vi "SQLite Example.vi"() -> ()   [LabVIEW 2011]
uses:
  State.ctl
  <vilib>/Analysis/NI_AALBase.lvlib
panel:
  out "Mean":dbl format="%0.2f"
  out "Failures":i32
  out "Voltage Waveform":dbl[](graph)
  # "Please refer to the readme in this project to make sure that the SQLite Engine is correctly installed on the real-time target"
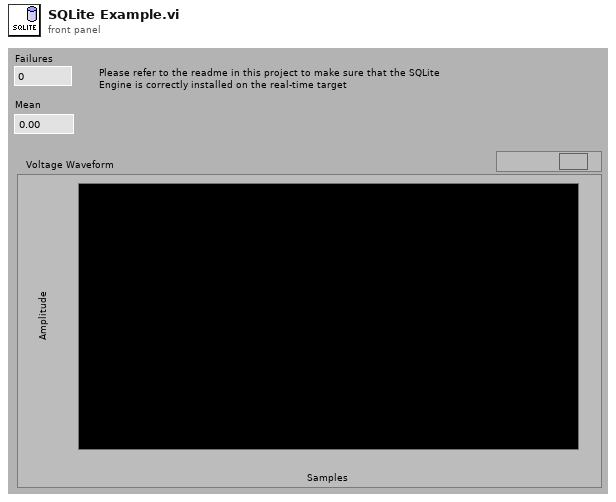
[diagram p1: front panel]
types:
  T1 = typedef "State.ctl" = enum16{"Empty Database", "Simulate Test", "Log DB", "Process DB", "Shutdown"}
  T2 = cluster{"RT State":T1, "Iteration":i32, "Record":cluster{"Iteration":i32, "Pass":bool, "Voltage":dbl, "log time":timestamp}}
  T3 = cluster{"Iteration":i32, "Pass":bool, "Voltage":dbl, "log time":timestamp}
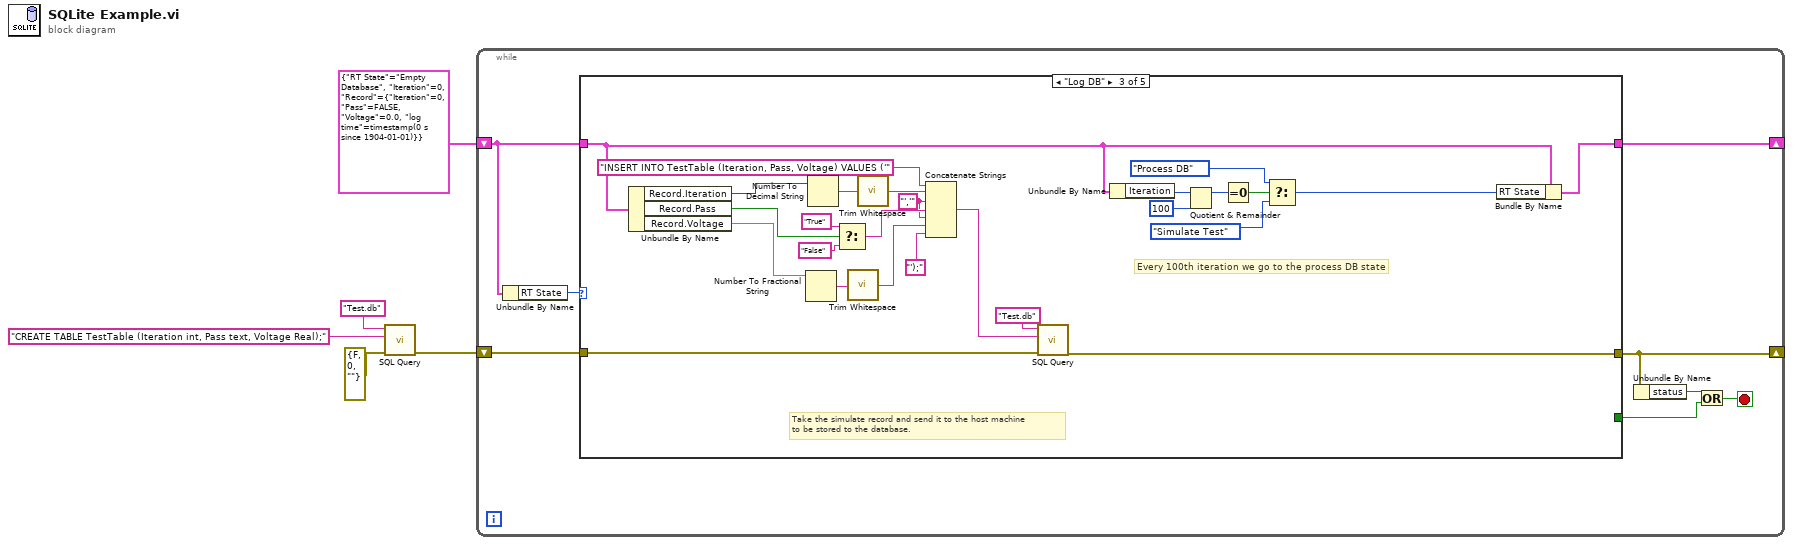
[diagram p0: block diagram]
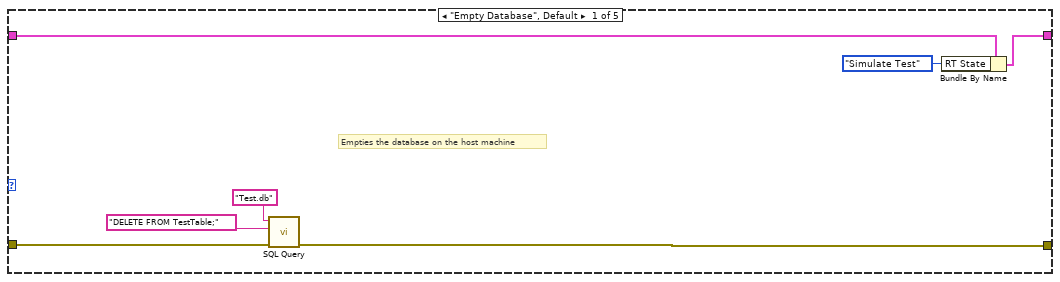
[diagram p2: hidden frame]
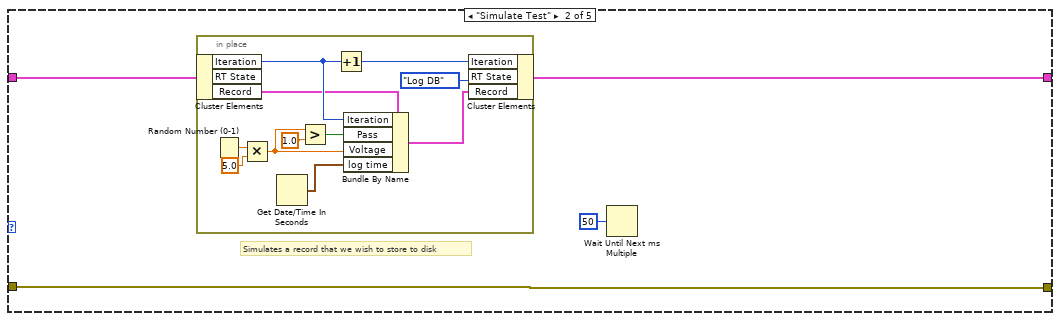
[diagram p3: hidden frame]
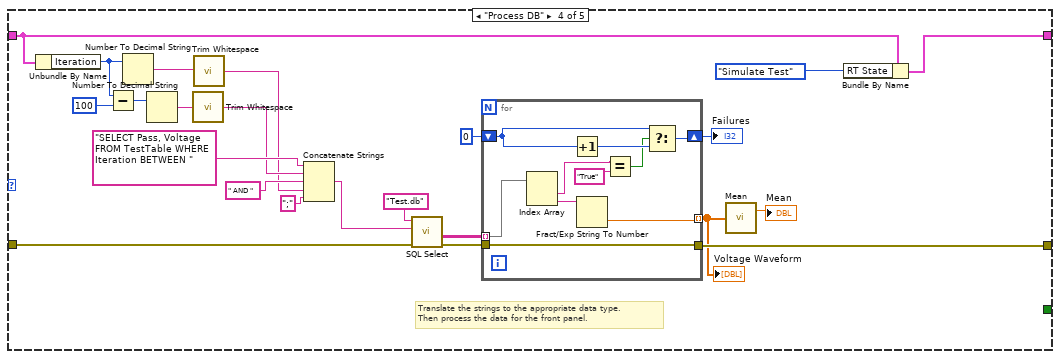
[diagram p4: hidden frame]
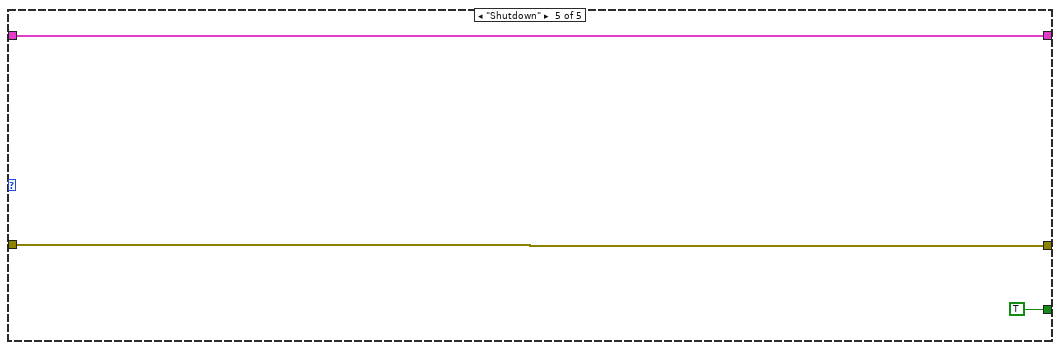
[diagram p5: hidden frame]
diagram:
  n1 = call "SQL Query.vi"("error in (no error)"=errorcluster {"status"=FALSE, "code"=0, "source"=""}, "SQL Query"="CREATE TABLE TestTable (Iteration int, Pass text, Voltage Real);", "Database File"="Test.db") -> ("error out"=w4:errorcluster)  [unwired: 6 in, 2 out]
  n2 = while {
    shift-right: [w13] -> _
    shift-left: T2 {"RT State"=enum."Empty Database", "Iteration"=0, "Record"={"Iteration"=0, "Pass"=FALSE, "Voltage"=0.0, "log time"=timestamp(0 s since 1904-01-01)}} -> [w12]
    shift-right: [w9] -> _
    shift-left: w4 -> [w10]
    stop <- w6 stop-if-true
    n3 = Unbundle By Name(w12) -> ("RT State"=w11:T1)
    n4 = case shown="\"Log DB\"" w11 {
      tunnel: [w14 w21 w51 w76 w95] -> w9
      tunnel: [_ _ _ _ TRUE] -> w7
      tunnel: w12 -> [w19 w23 w60 w71 w96]
      tunnel: [w20 w22 w53 w69 w96] -> w13
      tunnel: w10 -> [w17 w21 w52 w67 w95]
      frame "Empty Database", Default {
        # "Empties the database on the host machine"
        n5 = call "SQL Query.vi"("error in (no error)"=w17, "SQL Query"="DELETE FROM TestTable;", "Database File"="Test.db") -> ("error out"=w14:errorcluster)  [unwired: 6 in, 2 out]
        n6 = Bundle By Name(cluster=w19, "RT State"=State."Simulate Test") -> (w20:T2)
      }
      frame "Simulate Test" {
        # "Simulates a record that we wish to store to disk"
        n7 = in-place {
          n8 = in-place-cluster #1(w23) -> ("Iteration"=w27:i32, "Record"=w26:T3)  [unwired: 1 out]
          n9 = Random Number (0-1)() -> (number: 0 to 1=w35:dbl)
          n10 = Multiply(x=w35, y=5.0) -> (x*y=w29:dbl)
          n11 = Get Date/Time In Seconds() -> (seconds since 1Jan1904=w28:timestamp)
          n12 = Greater?(x=w29, y=1.0 ("x")) -> (0:w33:bool)
          n13 = Increment(x=w27) -> (x+1=w32:i32)
          n14 = Bundle By Name(cluster=w26, "Iteration"=w27, "Pass"=w33, "Voltage"=w29, "log time"=w28) -> (w31:T3)
          n15 = in-place-cluster #1("Iteration"=w32, "RT State"=State."Log DB", "Record"=w31) -> (w22:T2)
        }
        n16 = Wait Until Next ms Multiple(millisecond multiple=u32 50) -> ()  [unwired: 1 out]
      }
      frame "Log DB" {
        w36 = "','" ("string")
        # "Every 100th iteration we go to the process DB state"
        # "Take the simulate record and send it to the host machine\nto be stored to the database."
        n17 = Unbundle By Name(w60) -> ("Record.Iteration"=w50:i32, "Record.Pass"=w48:bool, "Record.Voltage"=w45:dbl)
        n18 = Number To Fractional String(number=w45) -> (F-format string=w44:string)  [unwired: 3 in]
        n19 = Number To Decimal String(number=w50) -> (decimal integer string=w49:string)  [unwired: 1 in]
        n20 = Select(t="True", s=w48, f="False") -> (s? t:f=w42:string)
        n21 = call <vilib>:"Trim Whitespace.vi"("string"=w44) -> ("trimmed string"=w41:string)  [unwired: 1 in]
        n22 = call <vilib>:"Trim Whitespace.vi"("string"=w49) -> ("trimmed string"=w43:string)  [unwired: 1 in]
        n23 = Concatenate Strings("INSERT INTO TestTable (Iteration, Pass, Voltage) VALUES ('" ("SQL Query"), w43, w36, w42, w36, w41, "');" ("string")) -> (w38:string)
        n24 = call "SQL Query.vi"("error in (no error)"=w52, "SQL Query"=w38, "Database File"="Test.db") -> ("error out"=w51:errorcluster)  [unwired: 6 in, 2 out]
        n25 = Unbundle By Name(w60) -> ("Iteration"=w56:i32)
        n26 = Quotient & Remainder(x=w56, y=100) -> (x-y*floor(x/y)=w58:i32)  [unwired: 1 out]
        n27 = Equal To 0?(x=w58) -> (x = 0?=w57:bool)
        n28 = Select(t=State."Process DB" ("RT State"), s=w57, f=State."Simulate Test" ("RT State")) -> (s? t:f=w61:T1)
        n29 = Bundle By Name(cluster=w60, "RT State"=w61) -> (w53:T2)
      }
      frame "Process DB" {
        # "Translate the strings to the appropriate data type.\nThen process the data for the front panel."
        n30 = Unbundle By Name(w71) -> ("Iteration"=w63:i32)
        n31 = Subtract(x=w63, y=100) -> (x-y=w82:i32)
        n32 = Number To Decimal String(number=w63) -> (decimal integer string=w84:string)  [unwired: 1 in]
        n33 = Number To Decimal String(number=w82) -> (decimal integer string=w81:string)  [unwired: 1 in]
        n34 = call <vilib>:"Trim Whitespace.vi"("string"=w81) -> ("trimmed string"=w79:string)  [unwired: 1 in]
        n35 = call <vilib>:"Trim Whitespace.vi"("string"=w84) -> ("trimmed string"=w77:string)  [unwired: 1 in]
        n36 = Concatenate Strings("SELECT Pass, Voltage FROM TestTable WHERE Iteration BETWEEN " ("Data"), w79, " AND " ("Data"), w77, ";" ("string")) -> (w62:string)
        n37 = call "SQL Select.vi"("error in (no error)"=w67, "Select Statement"=w62, "Database Name"="Test.db") -> ("error out"=w66:errorcluster, "Select Result"=w64:string[][])  [unwired: 5 in, 2 out]
        n38 = for {
          tunnel: w66 -> [w91]
          tunnel: [w91] -> w76
          tunnel: [w85] -> w72 mode=indexing
          shift-right: [w94] -> w73
          shift-left: 0 -> [w92]
          tunnel: w64 -> [w90] mode=indexing
          n39 = Index Array(array=w90) -> (element #1=w88:string, element #2=w86:string)  [unwired: 2 in]
          n40 = Increment(x=w92) -> (x+1=w93:i32)
          n41 = Fract/Exp String To Number(string=w86) -> (number=w85:dbl)  [unwired: 3 in, 1 out]
          n42 = Equal?(x=w88, y="True") -> (x = y?=w89:bool)
          n43 = Select(t=w92, s=w89, f=w93) -> (s? t:f=w94:i32)
        }
        "Failures" <- w73
        "Voltage Waveform" <- w72
        n44 = call <vilib>:"Mean.vi"("X"=w72) -> ("mean"=→"Mean":dbl)  [unwired: 1 out]
        n45 = Bundle By Name(cluster=w71, "RT State"=State."Simulate Test") -> (w69:T2)
      }
      frame "Shutdown" {
      }
    }
    n46 = Unbundle By Name(w9) -> ("status"=w8:bool)
    n47 = Or(x=w8, y=w7) -> (x .or. y?=w6:bool)
  }
